vi "氨氮插入数据.vi"(0 "database":string, 1 "data":T1 {"单位" items=["ug/L", "mg/L", "ppm", "mg/m3", "cm", "ppb", "ug/m3", "%", "nmol/mol", "umol/mol", "MPN/L", "MPN/100ml", "ng/m3", "NTU", "无量纲", "ms/cm", "us/cm"]}, 3 "SN":string, 5 "table":string, 7 "测量模式":T2(ring)=enum."水样测试", 9 "数据标记表":string(combo)="N", 11 "error in (no error)":errorcluster) -> (15 "error out":errorcluster)   [LabVIEW 2016, in "斯坦道氨氮.lvlib"]
uses:
  <vilib>/Utility/sysdir.llb/System Directory Type.ctl
  <vilib>/Utility/error.llb/DialogType.ctl
  <vilib>/addons/database/Auxilliary.llb/DB Tools Transaction.ctl
  <vilib>/addons/database/Auxilliary.llb/DB Tools Isolation Level.ctl
  <vilib>/addons/database/Connection.llb/DB Tools Open Connec (String).vi
  <vilib>/addons/database/Connection.llb/Conn Execute.vi
  <vilib>/addons/database/Recordset.llb/Rec Destroy - Connection.vi
  <vilib>/addons/database/Recordset.llb/Rec Fetch Recordset Data (R).vi
  <vilib>/addons/database/Connection.llb/Conn Transaction.vi
  <vilib>/addons/database/NI_Database_API.lvlib
panel:
  out "为空？":bool
  out "recordset data":variant[][](array[variant])
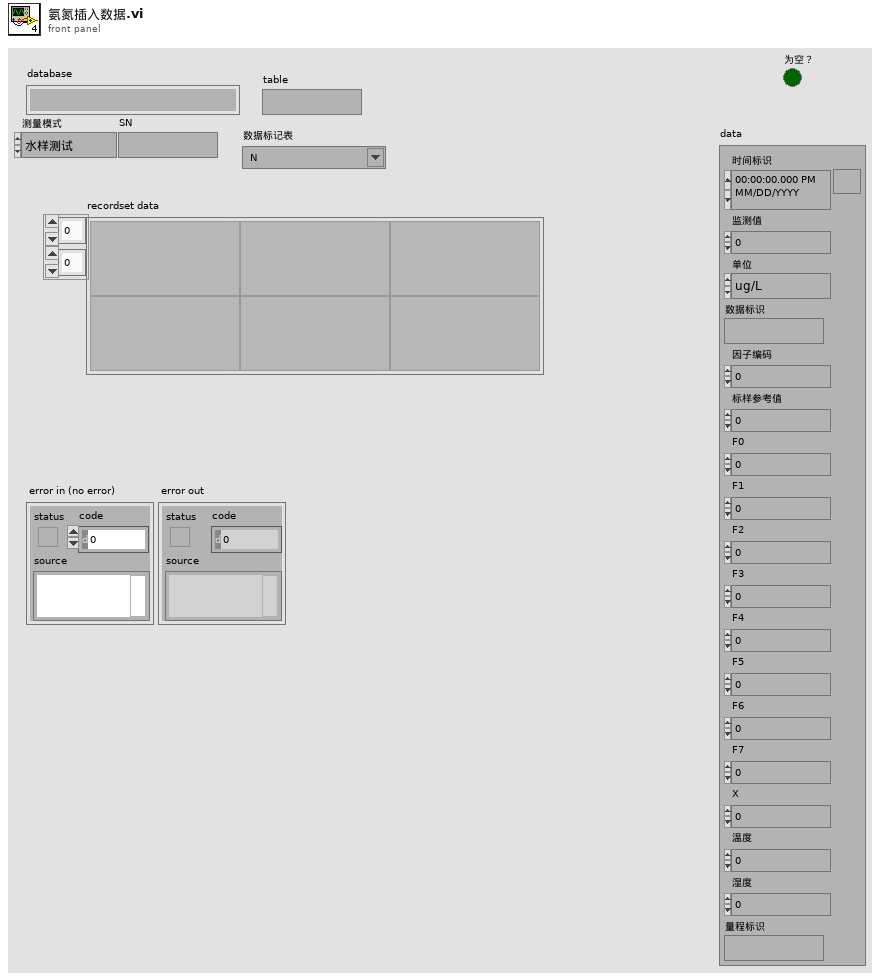
[diagram p1: front panel]
types:
  T1 = cluster{"时间标识":timestamp, "监测值":sgl, "单位":u16, "数据标识":string, "因子编码":u32, "标样参考值":sgl, "F0":sgl, "F1":sgl, "F2":sgl, "F3":sgl, "F4":sgl, "F5":sgl, "F6":sgl, "F7":sgl, "X":sgl, "温度":sgl, "湿度":sgl, "量程标识":string}
  T2 = enum16{"维护数据", "水样测试", "标样核查", "零点核查", "跨度核查", "空白测试", "平行样测试", "加标回收", "空白校准", "标样校准", "初始化（清洗）"}
  T3 = typedef "DialogType.ctl" = u16
  T4 = typedef "System Directory Type.ctl" = i32
  T5 = typedef "NI_Database_API.lvlib/Conn ObjectReference.ctl" = refnum<k1>
  T6 = typedef "NI_Database_API.lvlib/Rec ObjectReference.ctl" = refnum<k1>
  T7 = typedef "NI_Database_API.lvlib/DB Tools Transaction.ctl" = enum16{"begin", "commit", "rollback"}
  T8 = typedef "NI_Database_API.lvlib/DB Tools Isolation Level.ctl" = enum16{"chaos", "read uncommitted", "read committed", "repeatable read", "serializable"}
  T9 = cluster{"测量量程":dbl, "测量精度":dbl, "测量间隔":dbl, "消解温度":dbl, "消解时长":dbl, "空白校准时间":timestamp, "曲线截距":dbl, "曲线斜率":dbl, "测量检出限":dbl, "测量信号值":dbl, "线性相关系数":dbl, "二次多项式系数":dbl, "标样校准时间":timestamp, "稀释倍数":dbl, "三项式系数":dbl, "空白标定系数":dbl, "量程系数":dbl, "F0/ORPA":dbl, "F1/ORPB":dbl, "F2/ORPK":dbl, "F3":dbl, "F4":dbl, "F5":dbl, "F6":dbl, "F7":dbl, "X0/滴定数":dbl, "量程":dbl}
  T10 = cluster{"时间标识":timestamp, "测量模式":string, "数据类型":string, "监测值":sgl, "单位":string, "数据标识":string, "因子编码":string, "标样参考值":sgl, "F0":sgl, "F1":sgl, "F2":sgl, "F3":sgl, "F4":sgl, "F5":sgl, "F6":sgl, "F7":sgl, "X":sgl, "温度":sgl, "湿度":sgl, "量程标识":string, "SN":string, "Last Time":timestamp}
  T11 = cluster{"时间标识":timestamp, "设备":string, "日志信息":string}
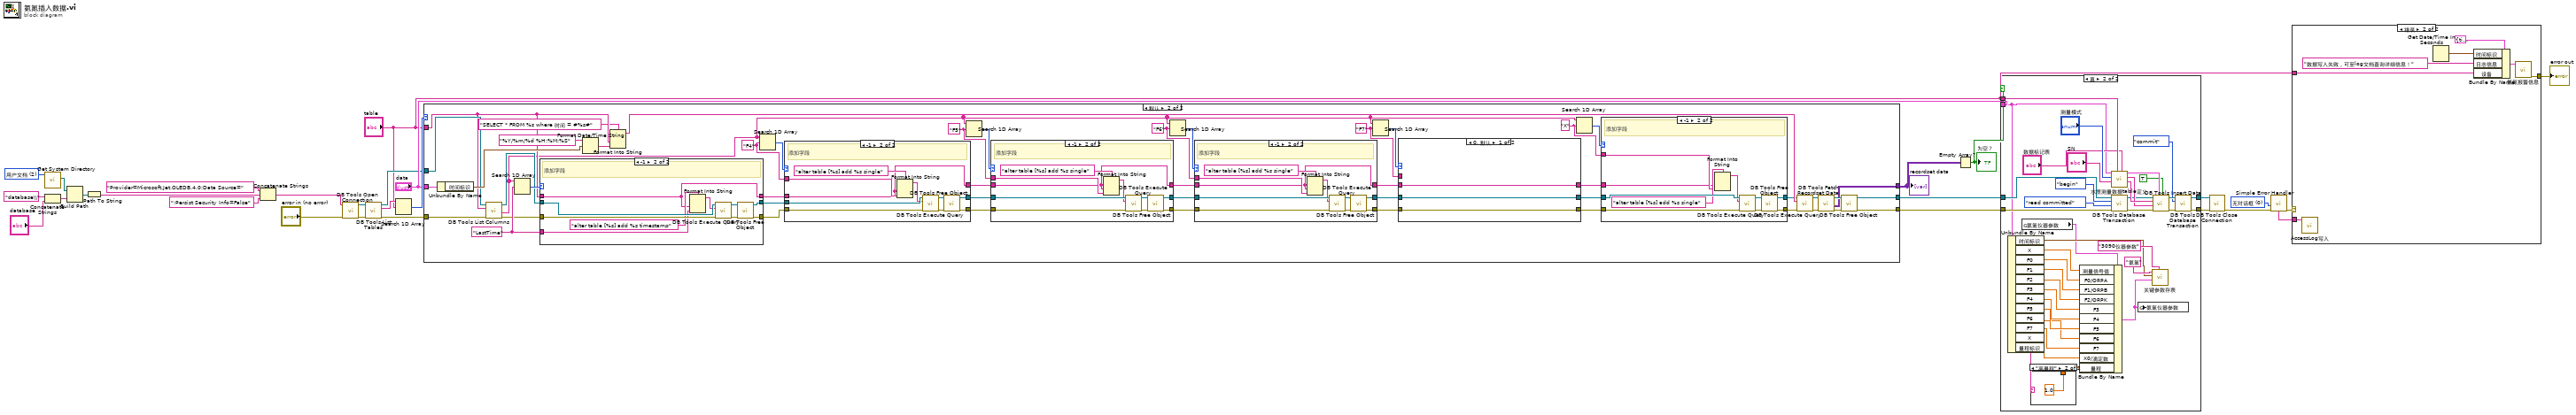
[diagram p0: block diagram]
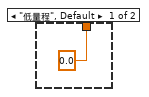
[diagram p4: hidden frame]
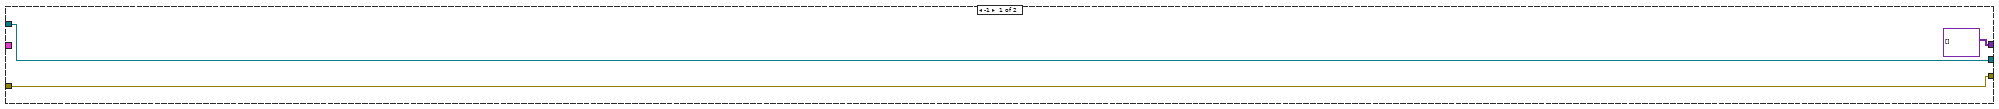
[diagram p5: hidden frame]
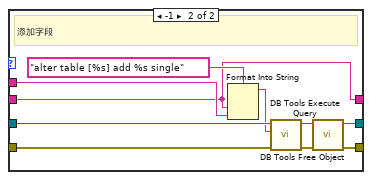
[diagram p7: hidden frame]
diagram:
  w5 = T3 0 items=["无对话框", "确定信息", "继续或停止信息", "确定信息＋警告", "继续/停止+警告"] ("type of dialog (OK msg:1)")
  w29 = T4 2 items=["用户目录"=0, "用户桌面"=1, "用户文档"=2, "用户应用程序数据"=3, "用户设置"=4, "用户临时目录"=5, "公共文档"=6, "公共应用程序数据"=7, "公共设置"=8, "公共缓存"=13, "系统核心库"=9, "系统安装库"=10, "应用程序文件"=11, "启动盘根目录"=12] ("system directory type")
  n1 = call <vilib>:"Get System Directory.vi"("system directory type"=w29) -> ("system directory"=w27:path)  [unwired: 10 in]
  n2 = Concatenate Strings("database\\" ("condition"), "database") -> (w21:string)
  n3 = Build Path(base path=w27, name or relative path=w21) -> (appended path=w26:path)
  n4 = Path To String(path=w26) -> (string=w25:string)
  n5 = Concatenate Strings("Provider=Microsoft.Jet.OLEDB.4.0;Data Source=" ("condition"), w25, ";Persist Security Info=False" ("condition")) -> (w23:string)
  n6 = call-poly <vilib>:"DB Tools Open Connection.vi"("error in (no error)"="error in (no error)", "connection information"=w23) -> ("error out"=w18:errorcluster, "connection reference"=w19:T5)  [unwired: 6 in]
  n7 = call <vilib>:"DB Tools List Tables.vi"("error in (no error)"=w18, "connection reference"=w19) -> ("error out"=w7:errorcluster, "tables"=w17:string[], "connection reference out"=w8:T5)  [unwired: 3 in]
  n8 = Search 1D Array(1D array=w17, element="table") -> (index of element=w16:i32)  [unwired: 1 in]
  n9 = case shown="默认" w16 {
    tunnel: [variant[][] [] ("recordset data") w77] -> w20
    tunnel: [w33 w76] -> w12
    tunnel: [w32 w75] -> w13
    tunnel: w8 -> [w33 w66]
    tunnel: w7 -> [w32 w65]
    tunnel: "table" -> [_ w64]
    tunnel: "data" -> [_ w70]
    frame -1 {
    }
    frame Default {
      w37 = "X" ("元素")
      w52 = "F7" ("元素")
      w53 = "F6" ("元素")
      w56 = "F5" ("元素")
      w57 = "F4" ("元素")
      w69 = "LastTime" ("元素")
      n10 = Unbundle By Name(w70) -> ("时间标识"=w73:timestamp)
      n11 = call <vilib>:"DB Tools List Columns.vi"("error in (no error)"=w65, "table"=w64, "connection reference"=w66) -> ("error out"=w68:errorcluster, "columns"=w39:string[], "connection reference out"=w61:T5)  [unwired: 1 in, 1 out]
      n12 = Search 1D Array(1D array=w39, element=w69) -> (index of element=w67:i32)  [unwired: 1 in]
      n13 = case shown="-1" w67 {
        tunnel: w61 -> [w148 w156]
        tunnel: w68 -> [w147 w155]
        tunnel: w69 -> [_ w153]
        tunnel: [w148 w151] -> w58
        tunnel: [w147 w150] -> w59
        tunnel: w64 -> [w146 w149]
        tunnel: [w146 w149] -> w60
        frame 0, Default {
        }
        frame -1 {
          # "添加字段"
          n14 = Format Into String(format string="alter table [%s] add %s timestamp", w149, w153) -> (resulting string=w152:string)  [unwired: 2 in, 1 out]
          n15 = call-poly <vilib>:"DB Tools Execute Query.vi"("error in (no error)"=w155, "SQL query"=w152, "connection reference"=w156) -> ("error out"=w157:errorcluster, "recordset reference"=w158:T6)  [unwired: 5 in]
          n16 = call-poly <vilib>:"DB Tools Free Object.vi"("error in (no error)"=w157, "recordset reference"=w158) -> ("error out"=w150:errorcluster, "connection reference"=w151:T5)  [unwired: 8 in]
        }
      }
      n17 = Format Date/Time String(time format string (%c)="%Y/%m/%d %H:%M:%S" ("时间格式字符串(%c)"), seconds (now)=w73) -> (date/time string=w71:string)  [unwired: 1 in]
      n18 = Format Into String(format string="SELECT * FROM %s where 时间 = #%s#" ("格式字符串"), w64, w71) -> (resulting string=w74:string)  [unwired: 2 in, 1 out]
      n19 = Search 1D Array(1D array=w39, element=w57) -> (index of element=w62:i32)  [unwired: 1 in]
      n20 = case shown="-1" w62 {
        tunnel: w58 -> [w135 w143]
        tunnel: w59 -> [w134 w142]
        tunnel: w57 -> [_ w140]
        tunnel: [w135 w138] -> w46
        tunnel: [w134 w137] -> w50
        tunnel: w60 -> [w133 w136]
        tunnel: [w133 w136] -> w45
        frame 0, Default {
        }
        frame -1 {
          # "添加字段"
          n21 = Format Into String(format string="alter table [%s] add %s single", w136, w140) -> (resulting string=w139:string)  [unwired: 2 in, 1 out]
          n22 = call-poly <vilib>:"DB Tools Execute Query.vi"("error in (no error)"=w142, "SQL query"=w139, "connection reference"=w143) -> ("error out"=w144:errorcluster, "recordset reference"=w145:T6)  [unwired: 5 in]
          n23 = call-poly <vilib>:"DB Tools Free Object.vi"("error in (no error)"=w144, "recordset reference"=w145) -> ("error out"=w137:errorcluster, "connection reference"=w138:T5)  [unwired: 8 in]
        }
      }
      n24 = Search 1D Array(1D array=w39, element=w56) -> (index of element=w55:i32)  [unwired: 1 in]
      n25 = case shown="-1" w55 {
        tunnel: w46 -> [w122 w130]
        tunnel: w50 -> [w121 w129]
        tunnel: w56 -> [_ w127]
        tunnel: [w122 w125] -> w44
        tunnel: [w121 w124] -> w49
        tunnel: w45 -> [w120 w123]
        tunnel: [w120 w123] -> w43
        frame 0, Default {
        }
        frame -1 {
          # "添加字段"
          n26 = Format Into String(format string="alter table [%s] add %s single", w123, w127) -> (resulting string=w126:string)  [unwired: 2 in, 1 out]
          n27 = call-poly <vilib>:"DB Tools Execute Query.vi"("error in (no error)"=w129, "SQL query"=w126, "connection reference"=w130) -> ("error out"=w131:errorcluster, "recordset reference"=w132:T6)  [unwired: 5 in]
          n28 = call-poly <vilib>:"DB Tools Free Object.vi"("error in (no error)"=w131, "recordset reference"=w132) -> ("error out"=w124:errorcluster, "connection reference"=w125:T5)  [unwired: 8 in]
        }
      }
      n29 = Search 1D Array(1D array=w39, element=w53) -> (index of element=w54:i32)  [unwired: 1 in]
      n30 = case shown="-1" w54 {
        tunnel: w44 -> [w109 w117]
        tunnel: w49 -> [w108 w116]
        tunnel: w53 -> [_ w114]
        tunnel: [w109 w112] -> w48
        tunnel: [w108 w111] -> w47
        tunnel: w43 -> [w107 w110]
        tunnel: [w107 w110] -> w42
        frame 0, Default {
        }
        frame -1 {
          # "添加字段"
          n31 = Format Into String(format string="alter table [%s] add %s single", w110, w114) -> (resulting string=w113:string)  [unwired: 2 in, 1 out]
          n32 = call-poly <vilib>:"DB Tools Execute Query.vi"("error in (no error)"=w116, "SQL query"=w113, "connection reference"=w117) -> ("error out"=w118:errorcluster, "recordset reference"=w119:T6)  [unwired: 5 in]
          n33 = call-poly <vilib>:"DB Tools Free Object.vi"("error in (no error)"=w118, "recordset reference"=w119) -> ("error out"=w111:errorcluster, "connection reference"=w112:T5)  [unwired: 8 in]
        }
      }
      n34 = Search 1D Array(1D array=w39, element=w52) -> (index of element=w51:i32)  [unwired: 1 in]
      n35 = case shown="0, 默认" w51 {
        tunnel: w48 -> [w96 w104]
        tunnel: w47 -> [w95 w103]
        tunnel: w52 -> [_ w101]
        tunnel: [w96 w99] -> w41
        tunnel: [w95 w98] -> w40
        tunnel: w42 -> [w94 w97]
        tunnel: [w94 w97] -> w36
        frame 0, Default {
        }
        frame -1 {
          # "添加字段"
          n36 = Format Into String(format string="alter table [%s] add %s single", w97, w101) -> (resulting string=w100:string)  [unwired: 2 in, 1 out]
          n37 = call-poly <vilib>:"DB Tools Execute Query.vi"("error in (no error)"=w103, "SQL query"=w100, "connection reference"=w104) -> ("error out"=w105:errorcluster, "recordset reference"=w106:T6)  [unwired: 5 in]
          n38 = call-poly <vilib>:"DB Tools Free Object.vi"("error in (no error)"=w105, "recordset reference"=w106) -> ("error out"=w98:errorcluster, "connection reference"=w99:T5)  [unwired: 8 in]
        }
      }
      n39 = Search 1D Array(1D array=w39, element=w37) -> (index of element=w38:i32)  [unwired: 1 in]
      n40 = case shown="-1" w38 {
        tunnel: w41 -> [w83 w91]
        tunnel: w40 -> [w82 w90]
        tunnel: w37 -> [_ w88]
        tunnel: [w83 w86] -> w35
        tunnel: [w82 w85] -> w34
        tunnel: w36 -> [_ w84]
        frame 0, Default {
        }
        frame -1 {
          # "添加字段"
          n41 = Format Into String(format string="alter table [%s] add %s single", w84, w88) -> (resulting string=w87:string)  [unwired: 2 in, 1 out]
          n42 = call-poly <vilib>:"DB Tools Execute Query.vi"("error in (no error)"=w90, "SQL query"=w87, "connection reference"=w91) -> ("error out"=w92:errorcluster, "recordset reference"=w93:T6)  [unwired: 5 in]
          n43 = call-poly <vilib>:"DB Tools Free Object.vi"("error in (no error)"=w92, "recordset reference"=w93) -> ("error out"=w85:errorcluster, "connection reference"=w86:T5)  [unwired: 8 in]
        }
      }
      n44 = call-poly <vilib>:"DB Tools Execute Query.vi"("error in (no error)"=w34, "SQL query"=w74, "connection reference"=w35) -> ("error out"=w78:errorcluster, "recordset reference"=w81:T6)  [unwired: 5 in]
      n45 = call-poly <vilib>:"DB Tools Fetch Recordset Data.vi"("error in (no error)"=w78, "recordset reference"=w81) -> ("error out"=w79:errorcluster, "recordset data"=w77:variant[][], "recordset reference out"=w80:T6)  [unwired: 3 in]
      n46 = call-poly <vilib>:"DB Tools Free Object.vi"("error in (no error)"=w79, "recordset reference"=w80) -> ("error out"=w75:errorcluster, "connection reference"=w76:T5)  [unwired: 8 in]
    }
  }
  "recordset data" <- w20
  n47 = Empty Array?(array=w20) -> (empty?=w14:bool)
  "为空？" <- w14
  n48 = case shown="真" w14 {
    tunnel: "table" -> [_ w197]
    tunnel: "data" -> [_ w166]
    tunnel: w13 -> [w159 w183]
    tunnel: w12 -> [w160 w195]
    tunnel: [w160 w186] -> w11
    tunnel: [w159 w184] -> w10
    frame False {
    }
    frame True {
      n49 = Unbundle By Name(w166) -> ("时间标识"=w163:timestamp, "X"=w178:sgl, "F0"=w177:sgl, "F1"=w176:sgl, "F2"=w175:sgl, "F3"=w174:sgl, "F4"=w173:sgl, "F5"=w172:sgl, "F6"=w171:sgl, "F7"=w170:sgl, "X"=w169:sgl, "量程标识"=w168:string)
      n50 = global read "氨氮断电保存全局变量.vi" "氨氮仪器参数"() -> (w162:T9)
      n51 = case shown="\"高量程\"" w168 {
        tunnel: [0.0 1.0] -> w167
        frame "低量程", Default {
        }
        frame "高量程" {
        }
      }
      n52 = Bundle By Name(cluster=w162, "测量信号值"=w178, "F0/ORPA"=w177, "F1/ORPB"=w176, "F2/ORPK"=w175, "F3"=w174, "F4"=w173, "F5"=w172, "F6"=w171, "F7"=w170, "X0/滴定数"=w169, "量程"=w167) -> (w161:T9)
      n53 = call "水质测量数据table定义.vi"("数据标记表"="数据标记表", "table 输入"=w197, "SN"="SN", "测量模式"="测量模式", "data"=w166) -> ("table 输出"=w192:string, "columns"=w191:string[], "data输出"=w194:T10)  [unwired: 4 in]
      n54 = call-poly <vilib>:"DB Tools Database Transaction.vi"("error in (no error)"=w183, "isolation level (chaos)"=DB_Tools_Isolation_Level."read committed", "operation (begin)"=DB_Tools_Transaction."begin", "connection reference"=w195) -> ("error out"=w182:errorcluster, "connection reference out"=w187:T5)  [unwired: 2 in]
      n55 = global write "氨氮断电保存全局变量.vi" "氨氮仪器参数"(w161) -> ()
      n56 = call "关键参数存表.vi"("table"="3090仪器参数", "仪器参数"=w161, "datatime"=w163, "仪器名称"="氨氮") -> ()  [unwired: 7 in, 1 out]
      n57 = call <vilib>:"DB Tools Insert Data.vi"("create table? (F)"=TRUE, "data"=w194, "error in (no error)"=w182, "columns"=w191, "table"=w192, "connection reference"=w187) -> ("error out"=w185:errorcluster, "connection reference out"=w190:T5)  [unwired: 4 in]
      n58 = call-poly <vilib>:"DB Tools Database Transaction.vi"("error in (no error)"=w185, "operation (begin)"=DB_Tools_Transaction."commit", "connection reference"=w190) -> ("error out"=w184:errorcluster, "connection reference out"=w186:T5)  [unwired: 3 in]
    }
  }
  n59 = call <vilib>:"DB Tools Close Connection.vi"("error in (no error)"=w10, "connection reference"=w11) -> ("error out"=w6:errorcluster)  [unwired: 5 in]
  n60 = call <vilib>:"Simple Error Handler.vi"("type of dialog (OK msg:1)"=w5, "error in (no error)"=w6) -> ("error out"=w4:errorcluster, "message"=w3:string)  [unwired: 3 in, 3 out]
  n61 = case shown="错误" w4 {
    tunnel: w3 -> [_ w200]
    tunnel: [_ w203] -> w2
    tunnel: "table" -> [_ w202]
    frame No Error {
    }
    frame Error {
      n62 = call "AccessLog写入.vi"("Log"=w200) -> ()  [unwired: 11 in]
      n63 = Get Date/Time In Seconds() -> (seconds since 1Jan1904=w205:timestamp)
      n64 = Bundle By Name(cluster=T11 {"时间标识"=timestamp(0 s since 1904-01-01), "设备"="", "日志信息"=""} ("data in"), "时间标识"=w205, "日志信息"="数据写入失败，可至log文档查询详细信息！", "设备"=w202) -> (w204:T11)
      n65 = call "氨氮报警信息.vi"("data in"=w204) -> ("error out"=w203:errorcluster)  [unwired: 10 in]
    }
  }
  "error out" <- w2
